vi "参数界面.vi"(8 "错误输入（无错误）":errorcluster, 10 "界面切换队列":refnum<queue>, 11 "VISA资源名称输入":refnum<visa-resource-name>) -> (0 "错误输出":errorcluster, 3 "VISA资源名称输出":refnum<visa-resource-name>)   [LabVIEW 2018]
panel:
  out "毫秒计时值":u32
  in  "枚举":T1(ring)
  in  "选项卡控件":enum32{"选项卡 1", "选项卡 2"}(tab)
  out "烧录座设定界面":bool
  out "极限参数界面":bool
  out "吸嘴偏移参数界面":bool
  out "读写R2481+R3禁用":bool
  out "DDT32534+R轴手动快速":dbl
  out "DDT32532+R轴手动慢速":dbl
  out "DDT32530+R轴减速时间":dbl
  out "DDT32528+R加速时间":dbl
  out "DDT32526+R轴最高速度":dbl
  out "DDT32524+R轴初始速度":dbl
  out "DDT32522+Z轴手动快速度":dbl
  out "DDT32520+Z轴手动慢速":dbl
  out "DDT32518+Z轴减速时间":dbl
  out "DDT32516+Z轴加速时间":dbl
  out "DDT32514+Z轴最高速度":dbl
  out "DDT32512+Z轴初始速度":dbl
  out "DDT32310+Y轴手动快速":dbl
  out "DDT32308+Y轴手动慢速":dbl
  out "DDT32306+Y轴减速时间":dbl
  out "DDT32304+Y轴加速时间":dbl
  out "DDT32302+Y轴最高速度":dbl
  out "DDT32300+Y轴初始速度":dbl
  out "DDT32510+X轴手动快速":dbl
  out "DDT32508+X轴手动慢速":dbl
  out "DDT32506+X轴减速时间":dbl
  out "DDT32504+X轴加速时间":dbl
  out "DDT32502+X轴最高速度":dbl
  out "DDT32500+X轴初始速度":dbl
  out "DDT32538+Z轴取料返回慢速长度":dbl
  out "DDT90356":dbl
  out "DDT90348":dbl
  out "自动界面":bool
  out "手动界面":bool
  out "参数界面":bool
  out "IO界面":bool
  out "产品界面":bool
  out "字符串":string
  out "DDT90352":dbl
  out "DDT90360":dbl
  out "DT1184":T2(ring)
  out "DDT32536+Z轴取料返回慢速":dbl
  in  "DT32730+枚举":enum16{"1拖2模式", "1拖4模式", "1拖8模式"}(ring)
  out "通讯周期":dbl
  # "X"
  # "Z1"
  # "XXXXX自动化设备有限公司"
  # "Z2"
  # "Y"
  # "速度参数"
  # "Z轴取料返回慢速长度"
  # "Z轴取料返回慢速"
  # "初始速度"
  # "最高速度"
  # "加速时间"
  # "减速时间"
  # "手动慢速"
  # "手动快速"
  # "X轴"
  # "Y轴"
  # "Z轴"
  # "R轴"
  # "选择1拖4或1拖8模式时，烧录座只能选择分开取放"
  # "烧录座模式请根据机器实际结构来更改，否则会出故障"
  # "烧录座模式"
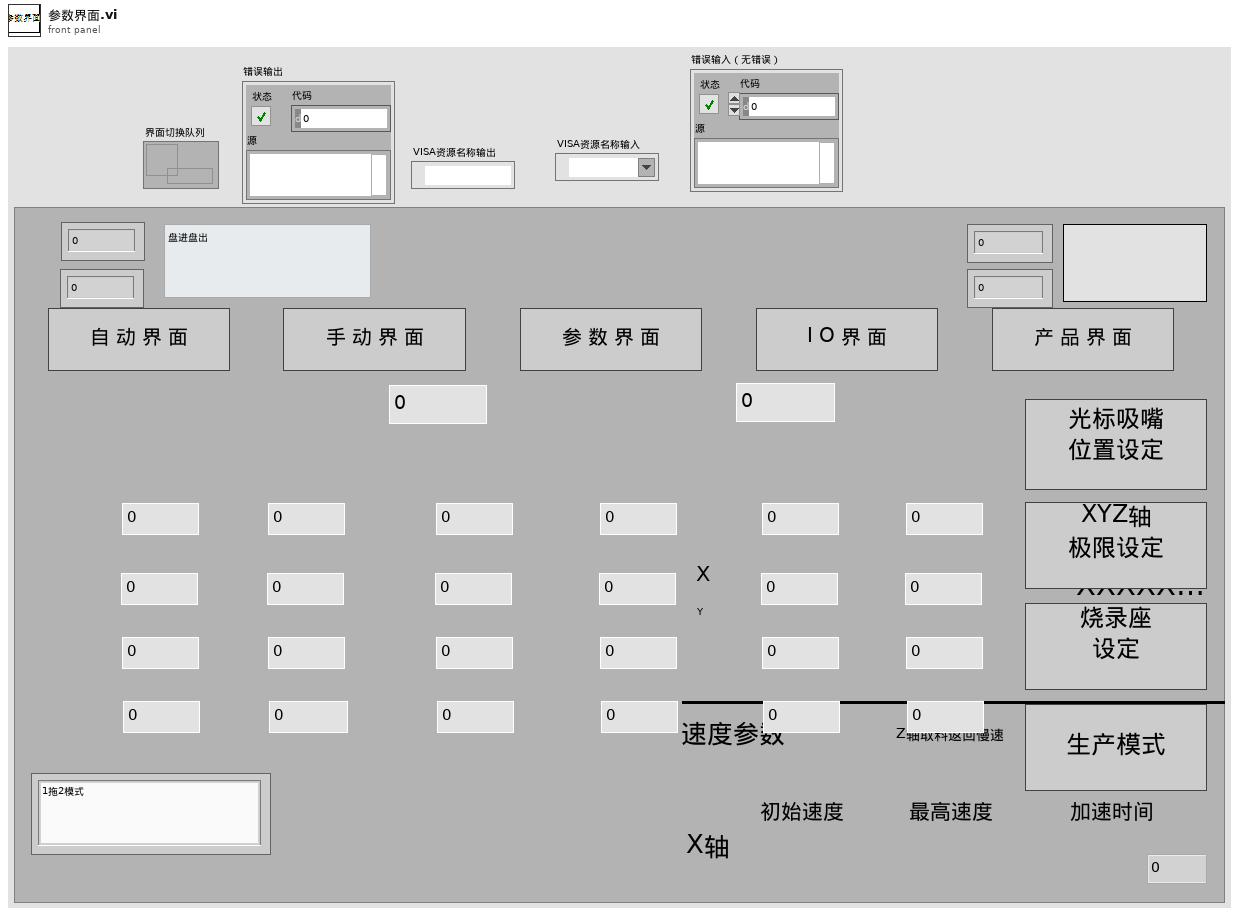
[diagram p1: front panel]
types:
  T1 = enum16{"读初始化", "读R3", "读R2481", "读DT32730+10", "读DDT32310+5", "读DDT32530+5", "读DDT32520+5", "读DDT32510+5", "读DDT32500+5", "读DDT32300+5", "读DDT90356", "读DT1184", "读DDT90348", ""}
  T2 = enum16{"盘进盘出", "卷进卷出", "盘进卷出", "管进盘出", "管进卷出", "卷进盘出", ""}
  T3 = enum8{"Enabled", "Disabled", "Disabled and Grayed Out"}
  T4 = typedef "数据簇.ctl" = cluster{"字符串":string, "数值":i32, "布尔":bool}
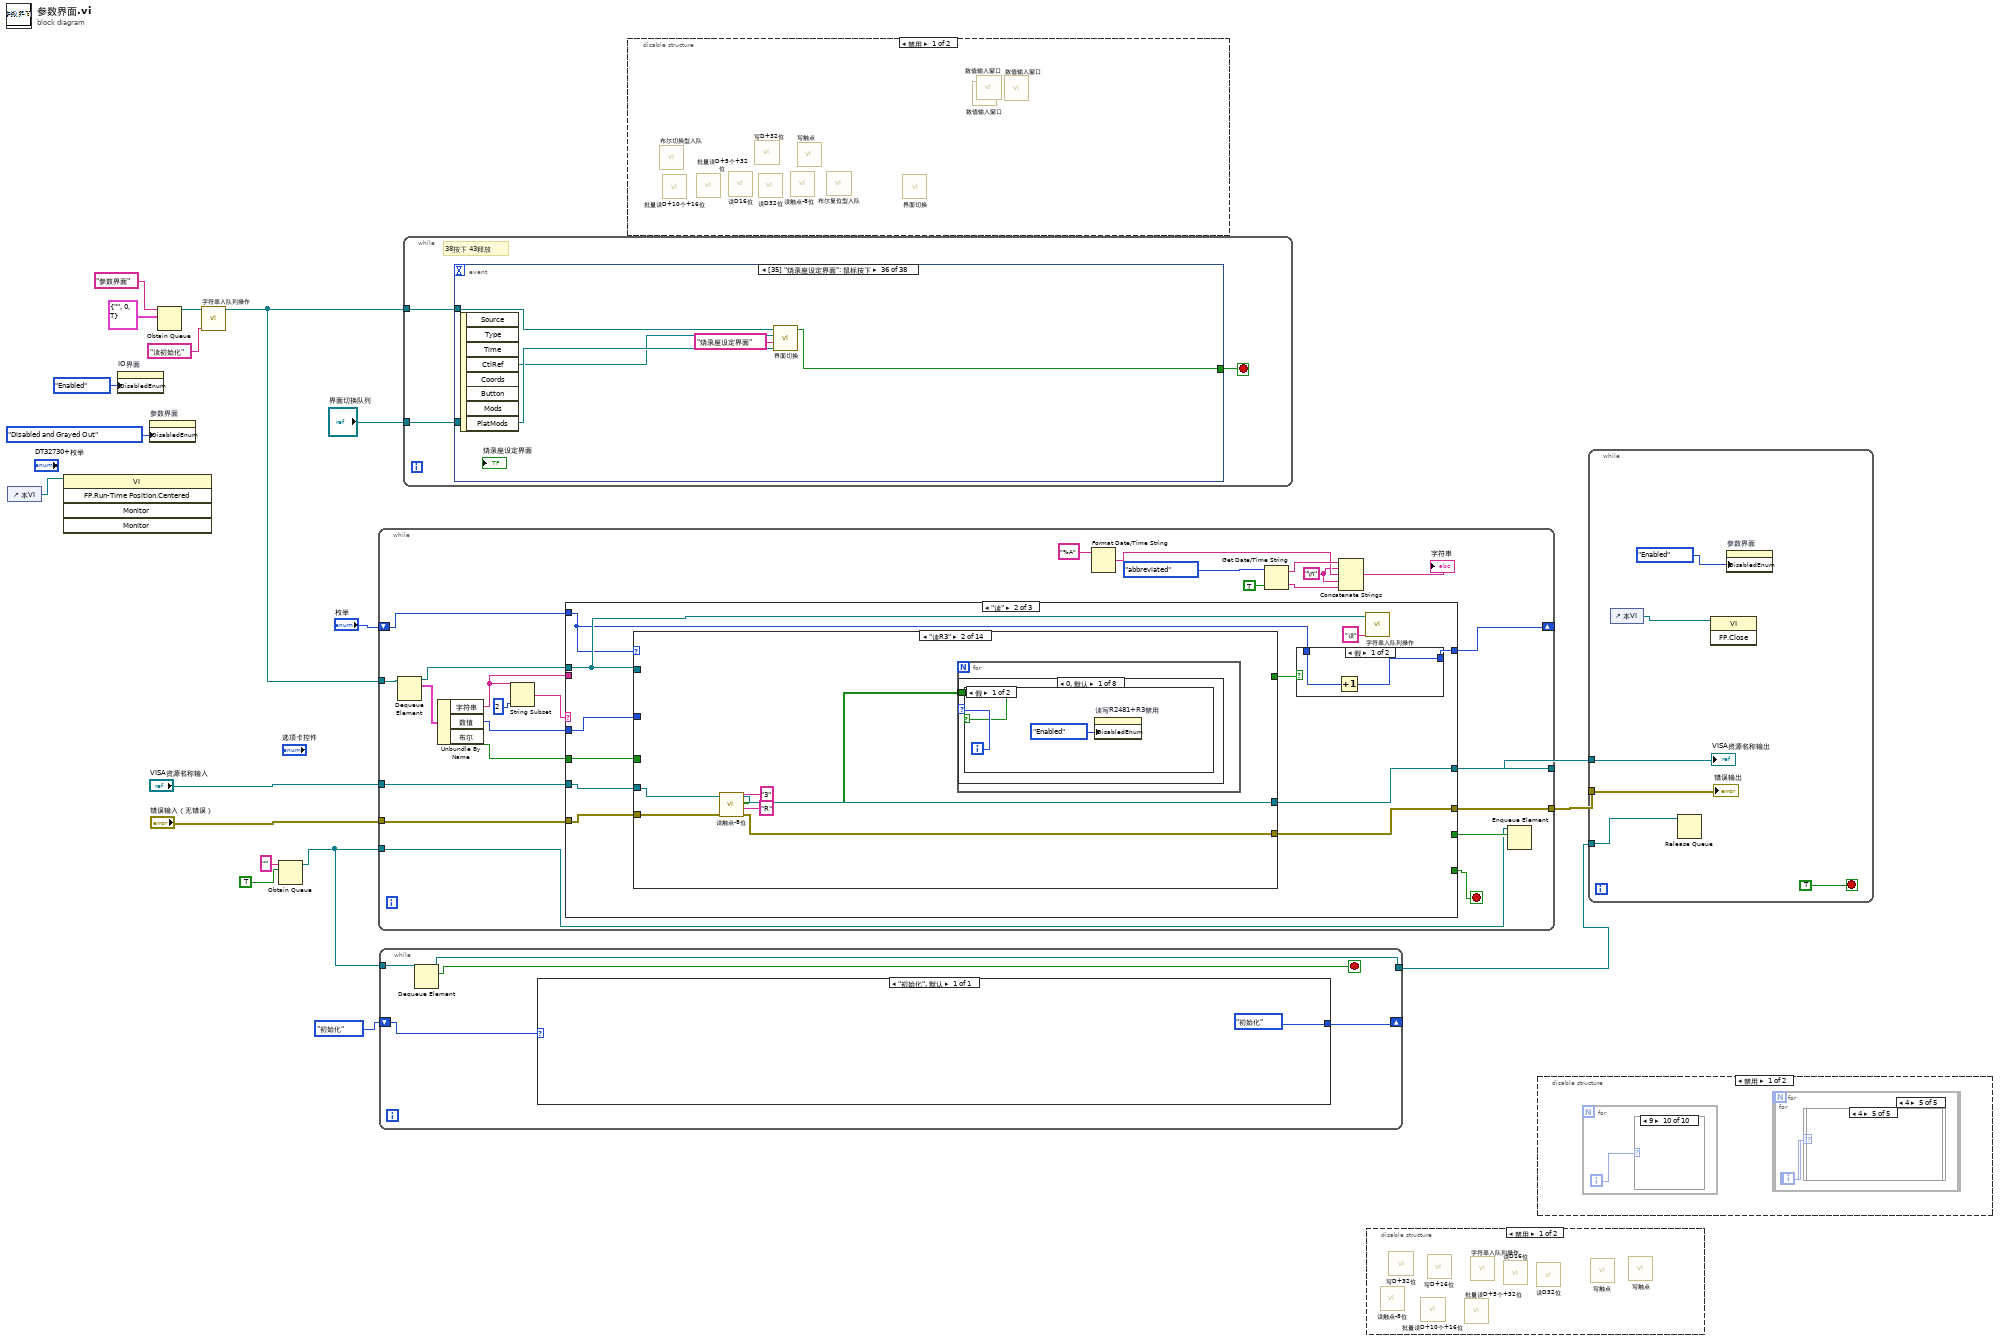
[diagram p0: block diagram]
diagram:
  n1 = control-ref of="本VI"() -> (w3:refnum<vi>)
  n2 = invoke class="VI" method="FP.Run-Time Position.Centered"(reference=w3) -> ()  [unwired: 4 in, 5 out]
  n3 = property on="IO界面" class="Bool"("DisabledEnum"=T3."Enabled" ("禁用")) -> ()  [unwired: 2 in, 2 out]
  n4 = property on="参数界面" class="Bool"("DisabledEnum"=T3."Disabled and Grayed Out" ("禁用")) -> ()  [unwired: 2 in, 2 out]
  n5 = Obtain Queue(name (unnamed)="参数界面" ("名称（未命名）"), element data type=T4 {"字符串"="", "数值"=0, "布尔"=TRUE}) -> (queue out=w12:refnum<queue>)  [unwired: 3 in, 2 out]
  n6 = call "字符串入队列操作.vi"("字符消息入队列"="读初始化", "界面切换队列"=w12) -> ("队列输出"=w4:refnum<queue>)  [unwired: 9 in]
  n7 = Obtain Queue(name (unnamed)="" ("名称（未命名）"), element data type=TRUE) -> (queue out=w7:refnum<queue>)  [unwired: 3 in, 2 out]
  n8 = while {
    tunnel: w4 -> [w40]
    tunnel: "VISA资源名称输入" -> [w33]
    tunnel: "错误输入（无错误）" -> [w32]
    tunnel: [w31] -> w14
    tunnel: [w30] -> w13
    shift-right: [w27] -> _
    shift-left: "枚举" -> [w28]
    tunnel: w7 -> [w20]
    stop <- w22 stop-if-true
    w24 = "\n"
    n9 = Dequeue Element(queue=w40) -> (queue out=w37:refnum<queue>, element=w39:T4)  [unwired: 2 in, 2 out]
    n10 = Unbundle By Name(w39) -> ("字符串"=w34:string, "数值"=w36:i32, "布尔"=w35:bool)
    n11 = String Subset(string=w34, length (rest)=2 ("长度（剩余）")) -> (substring=w38:string)  [unwired: 1 in]
    n12 = case shown="\"读\"" w38 {
      selector: w38 -> [w47 _ _]
      tunnel: w37 -> [_ w55 w231]
      tunnel: w36 -> [_ w62 w230]
      tunnel: w35 -> [_ w61 w229]
      tunnel: w34 -> [_ _ w223]
      tunnel: w33 -> [w46 w60 w228]
      tunnel: w32 -> [w45 w59 w227]
      tunnel: [w46 w58 w225] -> w31
      tunnel: [w45 w57 w224] -> w30
      tunnel: [_ _ w226] -> w22
      tunnel: w28 -> [_ w53 _]
      tunnel: [_ w52 _] -> w27
      tunnel: [_ _ w221] -> w21
      frame "", Default {
        n13 = Concatenate Strings("无对应消息分支**" ("消息"), w47, "**" ("字符串"), "读写状态机" ("字符串")) -> (w49:string)
        n14 = One Button Dialog(message=w49) -> ()  [unwired: 1 in, 1 out]
      }
      frame "读" {
        n15 = case shown="\"读R3\"" w53 {
          tunnel: w55 -> [_ _ _ _ _ _ _ _ _ _ _ _ _ _]
          tunnel: w62 -> [_ _ _ _ _ _ _ _ _ _ _ _ _ _]
          tunnel: w60 -> [w67 w74 w86 w95 w104 w113 w128 w141 w154 w167 w186 w195 w208 w220]
          tunnel: w59 -> [w66 w73 w85 w94 w103 w112 w127 w140 w153 w166 w185 w194 w207 w219]
          tunnel: [w67 w70 w82 w92 w101 w111 w126 w138 w151 w165 w184 w193 w206 w220] -> w58
          tunnel: [w66 w69 w81 w91 w100 w110 w125 w137 w150 w164 w183 w192 w205 w219] -> w57
          tunnel: w61 -> [_ _ _ _ _ _ _ _ _ _ _ _ _ _]
          tunnel: [_ _ _ _ _ _ _ _ _ _ _ _ _ TRUE] -> w54
          frame "读初始化" {
            n16 = Tick Count (ms)() -> (millisecond timer value=→"毫秒计时值":u32)
          }
          frame "读R3" {
            n17 = call "读触点-8位.vi"("error out"=w73, "触点类型"="R", "读取起始地址"="3", "VISA resource name out"=w74) -> ("error IO"=w69:errorcluster, "读取布尔数组"=w68:bool[], "VISA resource name out 2"=w70:refnum<visa-resource-name>)  [unwired: 4 in, 1 out]
            n18 = for {
              tunnel: w68 -> [w75] mode=indexing
              i -> [w76]
              n19 = case shown="0, 默认" w76 {
                tunnel: w75 -> [w77 _ _ _ _ _ _ _]
                frame 0, Default {
                  n20 = case shown="假" w77 {
                    frame False {
                      n21 = property on="读写R2481+R3禁用" class="Bool"("DisabledEnum"=T3."Enabled" ("禁用")) -> ()  [unwired: 2 in, 2 out]
                    }
                    frame True {
                      n22 = property on="读写R2481+R3禁用" class="Bool"("DisabledEnum"=T3."Disabled and Grayed Out" ("禁用")) -> ()  [unwired: 2 in, 2 out]
                    }
                  }
                }
                frame 1 {
                }
                frame 2 {
                }
                frame 3 {
                }
                frame 4 {
                }
                frame 5 {
                }
                frame 6 {
                }
                frame 7 {
                }
              }
            }
          }
          frame "读R2481" {
            n23 = call "读触点-8位.vi"("error out"=w85, "触点类型"="R", "读取起始地址"="2481", "VISA resource name out"=w86) -> ("error IO"=w81:errorcluster, "读取布尔数组"=w80:bool[], "VISA resource name out 2"=w82:refnum<visa-resource-name>)  [unwired: 4 in, 1 out]
            n24 = for {
              tunnel: w80 -> [w87] mode=indexing
              i -> [w88]
              n25 = case shown="0, 默认" w88 {
                tunnel: w87 -> [w89 _ _ _ _ _ _ _]
                frame 0, Default {
                  "读写R2481+R3禁用" <- w89
                }
                frame 1 {
                }
                frame 2 {
                }
                frame 3 {
                }
                frame 4 {
                }
                frame 5 {
                }
                frame 6 {
                }
                frame 7 {
                }
              }
            }
          }
          frame "读DT32730+10" {
            n26 = call "批量读D+10个+16位.vi"("error out"=w94, "读取D地址"=32730, "VISA resource name out"=w95) -> ("error IO"=w91:errorcluster, "数组"=w90:i32[], "VISA resource name out 2"=w92:refnum<visa-resource-name>)  [unwired: 5 in, 1 out]
            n27 = for {
              tunnel: w90 -> [w96] mode=indexing
              i -> [w97]
              n28 = case shown="0, 默认" w97 {
                tunnel: w96 -> [w98 _ _ _ _ _ _ _ _ _]
                frame 0, Default {
                  n29 = local write "DT32730+枚举"(w98) -> ()
                }
                frame 8 {
                }
                frame 9 {
                }
                frame 1 {
                }
                frame 2 {
                }
                frame 3 {
                }
                frame 4 {
                }
                frame 5 {
                }
                frame 6 {
                }
                frame 7 {
                }
              }
            }
          }
          frame "读DDT32310+5" {
            n30 = call "批量读D+5个+32位.vi"("error out"=w103, "读取D地址"=32310, "VISA resource name out"=w104) -> ("error IO"=w100:errorcluster, "数组"=w99:i32[], "VISA resource name out 2"=w101:refnum<visa-resource-name>)  [unwired: 5 in, 1 out]
            n31 = for {
              tunnel: w99 -> [w105] mode=indexing
              i -> [w106]
              n32 = case shown="0, 默认" w106 {
                tunnel: w105 -> [w107 _ _ _ _]
                frame 0, Default {
                  "DDT32310+Y轴手动快速" <- w107
                }
                frame 1 {
                }
                frame 2 {
                }
                frame 3 {
                }
                frame 4 {
                }
              }
            }
          }
          frame "读DDT32530+5" {
            n33 = call "批量读D+5个+32位.vi"("error out"=w112, "读取D地址"=32530, "VISA resource name out"=w113) -> ("error IO"=w110:errorcluster, "数组"=w108:i32[], "VISA resource name out 2"=w111:refnum<visa-resource-name>)  [unwired: 5 in, 1 out]
            n34 = for {
              tunnel: w108 -> [w114] mode=indexing
              i -> [w115]
              n35 = case shown="1" w115 {
                tunnel: w114 -> [w116 w117 w118 w119 w121]
                frame 0, Default {
                  "DDT32530+R轴减速时间" <- w116
                }
                frame 1 {
                  "DDT32532+R轴手动慢速" <- w117
                }
                frame 2 {
                  "DDT32534+R轴手动快速" <- w118
                }
                frame 3 {
                  "DDT32536+Z轴取料返回慢速" <- w119
                }
                frame 4 {
                  n36 = Divide(x=w121, y=100) -> (x/y=→"DDT32538+Z轴取料返回慢速长度":dbl)
                }
              }
            }
          }
          frame "读DDT32520+5" {
            n37 = call "批量读D+5个+32位.vi"("error out"=w127, "读取D地址"=32520, "VISA resource name out"=w128) -> ("error IO"=w125:errorcluster, "数组"=w123:i32[], "VISA resource name out 2"=w126:refnum<visa-resource-name>)  [unwired: 5 in, 1 out]
            n38 = for {
              tunnel: w123 -> [w129] mode=indexing
              i -> [w130]
              n39 = case shown="0, 默认" w130 {
                tunnel: w129 -> [w131 w132 w133 w134 w135]
                frame 0, Default {
                  "DDT32520+Z轴手动慢速" <- w131
                }
                frame 1 {
                  "DDT32522+Z轴手动快速度" <- w132
                }
                frame 2 {
                  "DDT32524+R轴初始速度" <- w133
                }
                frame 3 {
                  "DDT32526+R轴最高速度" <- w134
                }
                frame 4 {
                  "DDT32528+R加速时间" <- w135
                }
              }
            }
          }
          frame "读DDT32510+5" {
            n40 = call "批量读D+5个+32位.vi"("error out"=w140, "读取D地址"=32510, "VISA resource name out"=w141) -> ("error IO"=w137:errorcluster, "数组"=w136:i32[], "VISA resource name out 2"=w138:refnum<visa-resource-name>)  [unwired: 5 in, 1 out]
            n41 = for {
              tunnel: w136 -> [w142] mode=indexing
              i -> [w143]
              n42 = case shown="4" w143 {
                tunnel: w142 -> [w144 w145 w146 w147 w148]
                frame 0, Default {
                  "DDT32510+X轴手动快速" <- w144
                }
                frame 1 {
                  "DDT32512+Z轴初始速度" <- w145
                }
                frame 2 {
                  "DDT32514+Z轴最高速度" <- w146
                }
                frame 3 {
                  "DDT32516+Z轴加速时间" <- w147
                }
                frame 4 {
                  "DDT32518+Z轴减速时间" <- w148
                }
              }
            }
          }
          frame "读DDT32500+5" {
            n43 = call "批量读D+5个+32位.vi"("error out"=w153, "读取D地址"=32500, "VISA resource name out"=w154) -> ("error IO"=w150:errorcluster, "数组"=w149:i32[], "VISA resource name out 2"=w151:refnum<visa-resource-name>)  [unwired: 5 in, 1 out]
            n44 = for {
              tunnel: w149 -> [w155] mode=indexing
              i -> [w156]
              n45 = case shown="4" w156 {
                tunnel: w155 -> [w157 w158 w159 w160 w161]
                frame 0, Default {
                  "DDT32500+X轴初始速度" <- w157
                }
                frame 1 {
                  "DDT32502+X轴最高速度" <- w158
                }
                frame 2 {
                  "DDT32504+X轴加速时间" <- w159
                }
                frame 3 {
                  "DDT32506+X轴减速时间" <- w160
                }
                frame 4 {
                  "DDT32508+X轴手动慢速" <- w161
                }
              }
            }
          }
          frame "读DDT32300+5" {
            n46 = call "批量读D+5个+32位.vi"("error out"=w166, "读取D地址"=32300, "VISA resource name out"=w167) -> ("error IO"=w164:errorcluster, "数组"=w162:i32[], "VISA resource name out 2"=w165:refnum<visa-resource-name>)  [unwired: 5 in, 1 out]
            n47 = for {
              tunnel: w162 -> [w168] mode=indexing
              i -> [w169]
              n48 = case shown="0, 默认" w169 {
                tunnel: w168 -> [w170 w171 w172 w173 w174]
                frame 0, Default {
                  "DDT32300+Y轴初始速度" <- w170
                }
                frame 1 {
                  "DDT32302+Y轴最高速度" <- w171
                }
                frame 2 {
                  "DDT32304+Y轴加速时间" <- w172
                }
                frame 3 {
                  "DDT32306+Y轴减速时间" <- w173
                }
                frame 4 {
                  "DDT32308+Y轴手动慢速" <- w174
                }
              }
            }
          }
          frame "读DDT90356" {
            n49 = call "批量读D+5个+32位.vi"("error out"=w185, "读取D地址"=90356, "VISA resource name out"=w186) -> ("error IO"=w183:errorcluster, "数组"=w189:i32[], "VISA resource name out 2"=w184:refnum<visa-resource-name>)  [unwired: 5 in, 1 out]
            n50 = Index Array(array=w189, index #1=0 ("索引"), index #2=2 ("索引")) -> (element #1=w182:i32, element #2=w181:i32)
            n51 = To Double Precision Float(number=w182) -> (double precision float=w180:dbl)
            n52 = To Double Precision Float(number=w181) -> (double precision float=w177:dbl)
            n53 = Divide(x=w180, y=100.0) -> (x/y=→"DDT90356":dbl)
            n54 = Divide(x=w177, y=100.0) -> (x/y=→"DDT90360":dbl)
          }
          frame "读DT1184" {
            n55 = call "读D16位.vi"("error out"=w194, "读取D地址"=1184, "VISA resource name out"=w195) -> ("error IO"=w192:errorcluster, "数值"=→"DT1184":u32, "VISA resource name out 2"=w193:refnum<visa-resource-name>)  [unwired: 5 in, 1 out]
          }
          frame "读DDT90348" {
            n56 = call "批量读D+5个+32位.vi"("error out"=w207, "读取D地址"=90348, "VISA resource name out"=w208) -> ("error IO"=w205:errorcluster, "数组"=w212:i32[], "VISA resource name out 2"=w206:refnum<visa-resource-name>)  [unwired: 5 in, 1 out]
            n57 = Index Array(array=w212, index #1=0 ("索引"), index #2=2 ("索引")) -> (element #1=w204:i32, element #2=w203:i32)
            n58 = To Double Precision Float(number=w204) -> (double precision float=w202:dbl)
            n59 = To Double Precision Float(number=w203) -> (double precision float=w198:dbl)
            n60 = Divide(x=w202, y=100.0) -> (x/y=→"DDT90348":dbl)
            n61 = Divide(x=w198, y=100.0) -> (x/y=→"DDT90352":dbl)
          }
          frame "" {
            n62 = local read "毫秒计时值"() -> (w216:u32)
            n63 = Tick Count (ms)() -> (millisecond timer value=w217:u32)
            n64 = Subtract(x=w217, y=w216) -> (x-y=w215:u32)
            n65 = Divide(x=w215, y=u32 1000) -> (x/y=→"通讯周期":dbl)
          }
        }
        n66 = case shown="假" w54 {
          tunnel: w53 -> [w64 _]
          tunnel: [w63 _] -> w52
          frame False {
            n67 = Increment(x=w64) -> (x+1=w63:T1)
          }
          frame True {
          }
        }
        n68 = call "字符串入队列操作.vi"("字符消息入队列"="读", "界面切换队列"=w55) -> ()  [unwired: 9 in, 1 out]
      }
      frame "写" {
        n69 = call "状态匹配.vi"("输入状态"=w223) -> ("输出状态"=w222:string)  [unwired: 10 in]
        n70 = case shown="\"写DDT\"" w222 {
          selector: w222 -> [w234 _ _ _ _]
          tunnel: w231 -> [_ _ _ _ w274]
          tunnel: w230 -> [_ w240 w257 _ _]
          tunnel: w229 -> [_ _ _ w268 _]
          tunnel: w228 -> [w233 w250 w261 w273 w279]
          tunnel: w227 -> [w232 w249 w260 w272 w278]
          tunnel: [_ _ _ _ w277] -> w226
          tunnel: [w233 w248 w259 w271 w279] -> w225
          tunnel: [w232 w247 w258 w270 w278] -> w224
          tunnel: w223 -> [_ w239 w251 w262 _]
          tunnel: [_ _ _ _ w277] -> w221
          frame "", Default {
            n71 = Concatenate Strings("无对应消息分支**" ("消息"), w234, "**" ("字符串"), "写状态机" ("字符串")) -> (w238:string)
            n72 = One Button Dialog(message=w238) -> ()  [unwired: 1 in, 1 out]
          }
          frame "写DT" {
            n73 = String Length(string=w239) -> (length=w245:i32)
            n74 = Subtract(x=w245, y=4) -> (x-y=w243:i32)
            n75 = String Subset(string=w239, offset (0)=4 ("偏移量(0)"), length (rest)=w243) -> (substring=w242:string)
            n76 = Decimal String To Number(string=w242) -> (number=w241:i32)  [unwired: 2 in, 1 out]
            n77 = call "写D+16位.vi"("error out"=w249, "输入数值"=w240, "输入地址D"=w241, "VISA resource name out"=w250) -> ("error out 2"=w247:errorcluster, "VISA resource name out 2"=w248:refnum<visa-resource-name>)  [unwired: 3 in, 3 out]
          }
          frame "写DDT" {
            n78 = String Length(string=w251) -> (length=w255:i32)
            n79 = Subtract(x=w255, y=5) -> ()  [unwired: 1 out]
            n80 = String Subset(string=w251, offset (0)=5 ("偏移量(0)")) -> (substring=w252:string)  [unwired: 1 in]
            n81 = Decimal String To Number(string=w252) -> (number=w253:i32)  [unwired: 2 in, 1 out]
            n82 = call "写D+32位.vi"("error out"=w260, "输入数值"=w257, "输入地址D"=w253, "VISA resource name out"=w261) -> ("error out 2"=w258:errorcluster, "VISA resource name out 2"=w259:refnum<visa-resource-name>)  [unwired: 4 in, 2 out]
          }
          frame "写R" {
            n83 = String Length(string=w262) -> (length=w266:i32)
            n84 = Subtract(x=w266, y=3) -> (x-y=w264:i32)
            n85 = String Subset(string=w262, offset (0)=3 ("偏移量(0)"), length (rest)=w264) -> (substring=w263:string)
            n86 = call "写触点.vi"("布尔"=w268, "error out"=w272, "触点类型"="R", "写入起始地址"=w263, "VISA resource name out"=w273) -> ("error IO"=w270:errorcluster, "VISA resource name out 2"=w271:refnum<visa-resource-name>)  [unwired: 4 in, 1 out]
          }
          frame "写退出" {
            w277 = TRUE
            n87 = Flush Queue(queue=w274) -> (queue out=w275:refnum<queue>, error out=w276:errorcluster)  [unwired: 1 in, 1 out]
            n88 = Release Queue(queue=w275, error in (no error)=w276) -> ()  [unwired: 1 in, 3 out]
          }
        }
      }
    }
    n89 = Format Date/Time String(time format string (%c)="%A" ("时间格式字符串(%c)")) -> (date/time string=w25:string)  [unwired: 2 in]
    n90 = Get Date/Time String(date format (0)=enum16{"short", "long", "abbreviated"}."abbreviated" ("日期格式(0)"), want seconds? (F)=TRUE ("需要秒？(F)")) -> (date string=w42:string, time string=w23:string)  [unwired: 1 in]
    n91 = Concatenate Strings(w42, w24, w25, w24, w23) -> (→"字符串":string)
    n92 = Enqueue Element(queue=w20, element=w21) -> ()  [unwired: 2 in, 3 out]
  }
  n93 = while {
    shift-right: [w283] -> _
    shift-left: enum16{"初始化"}."初始化" -> [w284]
    tunnel: w7 -> [w282]
    tunnel: [w280] -> w6
    stop <- w281 stop-if-true
    n94 = Dequeue Element(queue=w282) -> (queue out=w280:refnum<queue>, element=w281:bool)  [unwired: 2 in, 2 out]
    n95 = case shown="\"初始化\", 默认" w284 {
      tunnel: [enum16{"初始化"}."初始化"] -> w283
      frame "初始化", Default {
      }
    }
  }
  n96 = while {
    tunnel: w4 -> [w287]
    tunnel: "界面切换队列" -> [w286]
    stop <- w288 stop-if-true
    # "38按下 43释放"
    n97 = event shown="[35] \"烧录座设定界面\": 鼠标按下" {
      selector: _ -> [_ _ _ _ _ _ _ _ _ _ _ _ _ _ _ _ _ _ _ _ _ _ _ _ _ _ _ _ _ _ _ _ _ _ _ _ _ _]
      dyn-events: _ -> [_ _ _ _ _ _ _ _ _ _ _ _ _ _ _ _ _ _ _ _ _ _ _ _ _ _ _ _ _ _ _ _ _ _ _ _ _ _]
      timeout: _ -> [_ _ _ _ _ _ _ _ _ _ _ _ _ _ _ _ _ _ _ _ _ _ _ _ _ _ _ _ _ _ _ _ _ _ _ _ _ _]
      tunnel: [w289 _ _ _ _ _ _ _ _ _ _ _ _ _ _ _ _ _ _ _ _ _ _ _ _ _ _ _ _ w509 w514 w523 w524 w529 w534 w539 _ w546] -> w288
      tunnel: w287 -> [w293 w297 w300 w308 w315 w324 w332 w340 w348 w356 w364 w372 w380 w388 w396 w404 w412 w420 w428 w436 w444 w452 w460 w468 w476 w484 w492 w500 w508 w513 w518 w522 w528 w533 w538 w543 _ w545]
      tunnel: w286 -> [w292 _ _ _ _ _ _ _ _ _ _ _ _ _ _ _ _ _ _ _ _ _ _ _ _ _ _ _ _ w512 w517 w521 w527 w532 w537 w542 _ w544]
      event "IO界面": Mouse Down {
        n98 = event-data() -> ("CtlRef"=w291:refnum<vi>)  [unwired: 1 in, 7 out]
        n99 = call "界面切换.vi"("界面切换队列输入"=w292, "切换界面名称输入"="IO界面", "Bool引用句柄"=w291, "状态转移输入"=w293) -> ("布尔"=w289:bool)  [unwired: 7 in]
      }
      event "读写R2481+R3禁用": Mouse Down {
        n100 = event-data() -> ("CtlRef"=w296:refnum<vi>)  [unwired: 1 in, 7 out]
        n101 = call "布尔切换型入队.vi"("字符串"="写R2481", "true启用入队"=TRUE, "控件引用"=w296, "消息入队列"=w297) -> ()  [unwired: 8 in]
      }
      event "DT32730+枚举": Value Change {
        n102 = event-data() -> ("NewVal"=w299:enum16{"1拖2模式", "1拖4模式", "1拖8模式"})  [unwired: 1 in, 5 out]
        n103 = call "字符串入队列操作.vi"("字符消息入队列"="写DT32730", "数值"=w299, "界面切换队列"=w300) -> ()  [unwired: 8 in, 1 out]
      }
      event "DDT32536+Z轴取料返回慢速": Mouse Down {
        n104 = event-data() -> ("CtlRef"=w301:refnum<vi>)  [unwired: 1 in, 7 out]
        n105 = call "数值输入窗口.vi"("消息入队"=w308, "字符串"="Z轴取料返回慢速", "字符消息入队列"="写DDT32536", "输入下限"=100.0, "输入上限"=60000.0, "转换比例"=u32 1, "数据类型"=enum16{"32位", "16位"}."32位", "控件引用"=w301) -> ()  [unwired: 5 in, 3 out]
      }
      event "DDT32538+Z轴取料返回慢速长度": Mouse Down {
        n106 = event-data() -> ("CtlRef"=w316:refnum<vi>)  [unwired: 1 in, 7 out]
        n107 = call "数值输入窗口.vi"("消息入队"=w315, "字符串"="Z轴取料返回慢速长度", "字符消息入队列"="写DDT32538", "输入下限"=0.0, "输入上限"=1000.0, "转换比例"=u32 100, "数据类型"=enum16{"32位", "16位"}."32位", "控件引用"=w316) -> ()  [unwired: 5 in, 3 out]
      }
      event "DDT32500+X轴初始速度": Mouse Down {
        n108 = event-data() -> ("CtlRef"=w317:refnum<vi>)  [unwired: 1 in, 7 out]
        n109 = call "数值输入窗口.vi"("消息入队"=w324, "字符串"="X轴初始速度", "字符消息入队列"="写DDT32500", "输入下限"=100.0, "输入上限"=1000.0, "转换比例"=u32 1, "数据类型"=enum16{"32位", "16位"}."32位", "控件引用"=w317) -> ()  [unwired: 5 in, 3 out]
      }
      event "DDT32502+X轴最高速度": Mouse Down {
        n110 = event-data() -> ("CtlRef"=w325:refnum<vi>)  [unwired: 1 in, 7 out]
        n111 = call "数值输入窗口.vi"("消息入队"=w332, "字符串"="X轴最高速度", "字符消息入队列"="写DDT32502", "输入下限"=100.0, "输入上限"=99000.0, "转换比例"=u32 1, "数据类型"=enum16{"32位", "16位"}."32位", "控件引用"=w325) -> ()  [unwired: 5 in, 3 out]
      }
      event "DDT32504+X轴加速时间": Mouse Down {
        n112 = event-data() -> ("CtlRef"=w334:refnum<vi>)  [unwired: 1 in, 7 out]
        n113 = call "数值输入窗口.vi"("消息入队"=w340, "字符串"="X轴加速时间", "字符消息入队列"="写DDT32504", "输入下限"=100.0, "输入上限"=99000.0, "转换比例"=u32 1, "数据类型"=enum16{"32位", "16位"}."32位", "控件引用"=w334) -> ()  [unwired: 5 in, 3 out]
      }
      event "DDT32506+X轴减速时间": Mouse Down {
        n114 = event-data() -> ("CtlRef"=w341:refnum<vi>)  [unwired: 1 in, 7 out]
        n115 = call "数值输入窗口.vi"("消息入队"=w348, "字符串"="X轴减速时间", "字符消息入队列"="写DDT32506", "输入下限"=100.0, "输入上限"=99000.0, "转换比例"=u32 1, "数据类型"=enum16{"32位", "16位"}."32位", "控件引用"=w341) -> ()  [unwired: 5 in, 3 out]
      }
      event "DDT32508+X轴手动慢速": Mouse Down {
        n116 = event-data() -> ("CtlRef"=w349:refnum<vi>)  [unwired: 1 in, 7 out]
        n117 = call "数值输入窗口.vi"("消息入队"=w356, "字符串"="X轴手动慢速", "字符消息入队列"="写DDT32508", "输入下限"=100.0, "输入上限"=99000.0, "转换比例"=u32 1, "数据类型"=enum16{"32位", "16位"}."32位", "控件引用"=w349) -> ()  [unwired: 5 in, 3 out]
      }
      event "DDT32510+X轴手动快速": Mouse Down {
        n118 = event-data() -> ("CtlRef"=w357:refnum<vi>)  [unwired: 1 in, 7 out]
        n119 = call "数值输入窗口.vi"("消息入队"=w364, "字符串"="X轴手动快速", "字符消息入队列"="写DDT32510", "输入下限"=100.0, "输入上限"=99000.0, "转换比例"=u32 1, "数据类型"=enum16{"32位", "16位"}."32位", "控件引用"=w357) -> ()  [unwired: 5 in, 3 out]
      }
      event "DDT32300+Y轴初始速度": Mouse Down {
        n120 = event-data() -> ("CtlRef"=w365:refnum<vi>)  [unwired: 1 in, 7 out]
        n121 = call "数值输入窗口.vi"("消息入队"=w372, "字符串"="Y轴初始速度", "字符消息入队列"="写DDT32300", "输入下限"=100.0, "输入上限"=1000.0, "转换比例"=u32 1, "数据类型"=enum16{"32位", "16位"}."32位", "控件引用"=w365) -> ()  [unwired: 5 in, 3 out]
      }
      event "DDT32302+Y轴最高速度": Mouse Down {
        n122 = event-data() -> ("CtlRef"=w373:refnum<vi>)  [unwired: 1 in, 7 out]
        n123 = call "数值输入窗口.vi"("消息入队"=w380, "字符串"="Y轴最高速度", "字符消息入队列"="写DDT32302", "输入下限"=100.0, "输入上限"=99000.0, "转换比例"=u32 1, "数据类型"=enum16{"32位", "16位"}."32位", "控件引用"=w373) -> ()  [unwired: 5 in, 3 out]
      }
      event "DDT32304+Y轴加速时间": Mouse Down {
        n124 = event-data() -> ("CtlRef"=w383:refnum<vi>)  [unwired: 1 in, 7 out]
        n125 = call "数值输入窗口.vi"("消息入队"=w388, "字符串"="Y轴加速时间", "字符消息入队列"="写DDT32304", "输入下限"=100.0, "输入上限"=99000.0, "转换比例"=u32 1, "数据类型"=enum16{"32位", "16位"}."32位", "控件引用"=w383) -> ()  [unwired: 5 in, 3 out]
      }
      event "DDT32306+Y轴减速时间": Mouse Down {
        n126 = event-data() -> ("CtlRef"=w389:refnum<vi>)  [unwired: 1 in, 7 out]
        n127 = call "数值输入窗口.vi"("消息入队"=w396, "字符串"="Y轴减速时间", "字符消息入队列"="写DDT32306", "输入下限"=100.0, "输入上限"=99000.0, "转换比例"=u32 1, "数据类型"=enum16{"32位", "16位"}."32位", "控件引用"=w389) -> ()  [unwired: 5 in, 3 out]
      }
      event "DDT32308+Y轴手动慢速": Mouse Down {
        n128 = event-data() -> ("CtlRef"=w397:refnum<vi>)  [unwired: 1 in, 7 out]
        n129 = call "数值输入窗口.vi"("消息入队"=w404, "字符串"="Y轴手动慢速", "字符消息入队列"="写DDT32308", "输入下限"=100.0, "输入上限"=99000.0, "转换比例"=u32 1, "数据类型"=enum16{"32位", "16位"}."32位", "控件引用"=w397) -> ()  [unwired: 5 in, 3 out]
      }
      event "DDT32310+Y轴手动快速": Mouse Down {
        n130 = event-data() -> ("CtlRef"=w405:refnum<vi>)  [unwired: 1 in, 7 out]
        n131 = call "数值输入窗口.vi"("消息入队"=w412, "字符串"="Y轴手动快速", "字符消息入队列"="写DDT32310", "输入下限"=100.0, "输入上限"=99000.0, "转换比例"=u32 1, "数据类型"=enum16{"32位", "16位"}."32位", "控件引用"=w405) -> ()  [unwired: 5 in, 3 out]
      }
      event "DDT32512+Z轴初始速度": Mouse Down {
        n132 = event-data() -> ("CtlRef"=w413:refnum<vi>)  [unwired: 1 in, 7 out]
        n133 = call "数值输入窗口.vi"("消息入队"=w420, "字符串"="Z轴初始速度", "字符消息入队列"="写DDT32512", "输入下限"=100.0, "输入上限"=1000.0, "转换比例"=u32 1, "数据类型"=enum16{"32位", "16位"}."32位", "控件引用"=w413) -> ()  [unwired: 5 in, 3 out]
      }
      event "DDT32514+Z轴最高速度": Mouse Down {
        n134 = event-data() -> ("CtlRef"=w421:refnum<vi>)  [unwired: 1 in, 7 out]
        n135 = call "数值输入窗口.vi"("消息入队"=w428, "字符串"="Z轴最高速度", "字符消息入队列"="写DDT32514", "输入下限"=100.0, "输入上限"=9900.0, "转换比例"=u32 1, "数据类型"=enum16{"32位", "16位"}."32位", "控件引用"=w421) -> ()  [unwired: 5 in, 3 out]
      }
      event "DDT32516+Z轴加速时间": Mouse Down {
        n136 = event-data() -> ("CtlRef"=w429:refnum<vi>)  [unwired: 1 in, 7 out]
        n137 = call "数值输入窗口.vi"("消息入队"=w436, "字符串"="Z轴加速时间", "字符消息入队列"="写DDT32516", "输入下限"=100.0, "输入上限"=99000.0, "转换比例"=u32 1, "数据类型"=enum16{"32位", "16位"}."32位", "控件引用"=w429) -> ()  [unwired: 5 in, 3 out]
      }
      event "DDT32518+Z轴减速时间": Mouse Down {
        n138 = event-data() -> ("CtlRef"=w437:refnum<vi>)  [unwired: 1 in, 7 out]
        n139 = call "数值输入窗口.vi"("消息入队"=w444, "字符串"="Z轴减速时间", "字符消息入队列"="写DDT32518", "输入下限"=100.0, "输入上限"=99000.0, "转换比例"=u32 1, "数据类型"=enum16{"32位", "16位"}."32位", "控件引用"=w437) -> ()  [unwired: 5 in, 3 out]
      }
      event "DDT32520+Z轴手动慢速": Mouse Down {
        n140 = event-data() -> ("CtlRef"=w445:refnum<vi>)  [unwired: 1 in, 7 out]
        n141 = call "数值输入窗口.vi"("消息入队"=w452, "字符串"="Z轴手动慢速", "字符消息入队列"="写DDT32520", "输入下限"=100.0, "输入上限"=99000.0, "转换比例"=u32 1, "数据类型"=enum16{"32位", "16位"}."32位", "控件引用"=w445) -> ()  [unwired: 5 in, 3 out]
      }
      event "DDT32522+Z轴手动快速度": Mouse Down {
        n142 = event-data() -> ("CtlRef"=w453:refnum<vi>)  [unwired: 1 in, 7 out]
        n143 = call "数值输入窗口.vi"("消息入队"=w460, "字符串"="Z轴手动快速", "字符消息入队列"="写DDT32522", "输入下限"=100.0, "输入上限"=99900.0, "转换比例"=u32 1, "数据类型"=enum16{"32位", "16位"}."32位", "控件引用"=w453) -> ()  [unwired: 5 in, 3 out]
      }
      event "DDT32524+R轴初始速度": Mouse Down {
        n144 = event-data() -> ("CtlRef"=w461:refnum<vi>)  [unwired: 1 in, 7 out]
        n145 = call "数值输入窗口.vi"("消息入队"=w468, "字符串"="R轴初始速度", "字符消息入队列"="写DDT32524", "输入下限"=100.0, "输入上限"=1000.0, "转换比例"=u32 1, "数据类型"=enum16{"32位", "16位"}."32位", "控件引用"=w461) -> ()  [unwired: 5 in, 3 out]
      }
      event "DDT32526+R轴最高速度": Mouse Down {
        n146 = event-data() -> ("CtlRef"=w469:refnum<vi>)  [unwired: 1 in, 7 out]
        n147 = call "数值输入窗口.vi"("消息入队"=w476, "字符串"="R轴最高速度", "字符消息入队列"="写DDT32526", "输入下限"=100.0, "输入上限"=9900.0, "转换比例"=u32 1, "数据类型"=enum16{"32位", "16位"}."32位", "控件引用"=w469) -> ()  [unwired: 5 in, 3 out]
      }
      event "DDT32528+R加速时间": Mouse Down {
        n148 = event-data() -> ("CtlRef"=w477:refnum<vi>)  [unwired: 1 in, 7 out]
        n149 = call "数值输入窗口.vi"("消息入队"=w484, "字符串"="R轴加速时间", "字符消息入队列"="写DDT32528", "输入下限"=100.0, "输入上限"=99900.0, "转换比例"=u32 1, "数据类型"=enum16{"32位", "16位"}."32位", "控件引用"=w477) -> ()  [unwired: 5 in, 3 out]
      }
      event "DDT32530+R轴减速时间": Mouse Down {
        n150 = event-data() -> ("CtlRef"=w487:refnum<vi>)  [unwired: 1 in, 7 out]
        n151 = call "数值输入窗口.vi"("消息入队"=w492, "字符串"="R轴减速时间", "字符消息入队列"="写DDT32530", "输入下限"=100.0, "输入上限"=99000.0, "转换比例"=u32 1, "数据类型"=enum16{"32位", "16位"}."32位", "控件引用"=w487) -> ()  [unwired: 5 in, 3 out]
      }
      event "DDT32532+R轴手动慢速": Mouse Down {
        n152 = event-data() -> ("CtlRef"=w495:refnum<vi>)  [unwired: 1 in, 7 out]
        n153 = call "数值输入窗口.vi"("消息入队"=w500, "字符串"="R轴手动慢速", "字符消息入队列"="写DDT32532", "输入下限"=100.0, "输入上限"=99000.0, "转换比例"=u32 1, "数据类型"=enum16{"32位", "16位"}."32位", "控件引用"=w495) -> ()  [unwired: 5 in, 3 out]
      }
      event "DDT32534+R轴手动快速": Mouse Down {
        n154 = event-data() -> ("CtlRef"=w501:refnum<vi>)  [unwired: 1 in, 7 out]
        n155 = call "数值输入窗口.vi"("消息入队"=w508, "字符串"="R轴手动快速", "字符消息入队列"="写DDT32534", "输入下限"=100.0, "输入上限"=99900.0, "转换比例"=u32 1, "数据类型"=enum16{"32位", "16位"}."32位", "控件引用"=w501) -> ()  [unwired: 5 in, 3 out]
      }
      event "参数界面": Mouse Down {
        n156 = event-data() -> ("CtlRef"=w511:refnum<vi>)  [unwired: 1 in, 7 out]
        n157 = call "界面切换.vi"("界面切换队列输入"=w512, "切换界面名称输入"="参数界面", "Bool引用句柄"=w511, "状态转移输入"=w513) -> ("布尔"=w509:bool)  [unwired: 7 in]
      }
      event "产品界面": Mouse Down {
        n158 = event-data() -> ("CtlRef"=w516:refnum<vi>)  [unwired: 1 in, 7 out]
        n159 = call "界面切换.vi"("界面切换队列输入"=w517, "切换界面名称输入"="产品界面", "Bool引用句柄"=w516, "状态转移输入"=w518) -> ("布尔"=w514:bool)  [unwired: 7 in]
      }
      event "手动界面": Mouse Down {
        n160 = event-data() -> ("CtlRef"=w520:refnum<vi>)  [unwired: 1 in, 7 out]
        n161 = call "界面切换.vi"("界面切换队列输入"=w521, "切换界面名称输入"="手动界面", "Bool引用句柄"=w520, "状态转移输入"=w522) -> ("布尔"=w523:bool)  [unwired: 7 in]
      }
      event "自动界面": Mouse Down {
        n162 = event-data() -> ("CtlRef"=w526:refnum<vi>)  [unwired: 1 in, 7 out]
        n163 = call "界面切换.vi"("界面切换队列输入"=w527, "切换界面名称输入"="自动界面", "Bool引用句柄"=w526, "状态转移输入"=w528) -> ("布尔"=w524:bool)  [unwired: 7 in]
      }
      event "吸嘴偏移参数界面": Mouse Down {
        n164 = event-data() -> ("CtlRef"=w530:refnum<vi>)  [unwired: 1 in, 7 out]
        n165 = call "界面切换.vi"("界面切换队列输入"=w532, "切换界面名称输入"="吸嘴偏移参数界面", "Bool引用句柄"=w530, "状态转移输入"=w533) -> ("布尔"=w529:bool)  [unwired: 7 in]
      }
      event "极限参数界面": Mouse Down {
        n166 = event-data() -> ("CtlRef"=w536:refnum<vi>)  [unwired: 1 in, 7 out]
        n167 = call "界面切换.vi"("界面切换队列输入"=w537, "切换界面名称输入"="极限参数界面", "Bool引用句柄"=w536, "状态转移输入"=w538) -> ("布尔"=w534:bool)  [unwired: 7 in]
      }
      event "烧录座设定界面": Mouse Down {
        n168 = event-data() -> ("CtlRef"=w541:refnum<vi>)  [unwired: 1 in, 7 out]
        n169 = call "界面切换.vi"("界面切换队列输入"=w542, "切换界面名称输入"="烧录座设定界面", "Bool引用句柄"=w541, "状态转移输入"=w543) -> ("布尔"=w539:bool)  [unwired: 7 in]
      }
      event Timeout {
        n170 = event-data() -> ()  [unwired: 1 in, 3 out]
      }
      event Panel Close? {
        n171 = event-data() -> ()  [unwired: 1 in, 4 out]
        n172 = Two Button Dialog(message="确定退出程序？" ("消息")) -> (T button?=w547:bool)  [unwired: 2 in]
        n173 = case shown="真" w547 {
          tunnel: [_ TRUE] -> w546
          tunnel: w545 -> [_ w552]
          tunnel: w544 -> [_ w551]
          frame False {
          }
          frame True {
            n174 = call "字符串入队列操作.vi"("字符消息入队列"="退出", "界面切换队列"=w551) -> ()  [unwired: 9 in, 1 out]
            n175 = call "字符串入队列操作.vi"("字符消息入队列"="写退出", "界面切换队列"=w552) -> ()  [unwired: 9 in, 1 out]
          }
        }
        n176 = event-data("Discard?"=TRUE ("放弃？")) -> ()  [unwired: 1 in, 1 out]
      }
    }
  }
  n177 = disable-structure shown="禁用" {
    frame Disabled {
      n178 = call "布尔切换型入队.vi"() -> ()  [unwired: 12 in]
      n179 = call "批量读D+10个+16位.vi"() -> ()  [unwired: 8 in, 4 out]
      n180 = call "批量读D+5个+32位.vi"() -> ()  [unwired: 8 in, 4 out]
      n181 = call "读D16位.vi"() -> ()  [unwired: 8 in, 4 out]
      n182 = call "写D+32位.vi"() -> ()  [unwired: 8 in, 4 out]
      n183 = call "读D32位.vi"() -> ()  [unwired: 9 in, 3 out]
      n184 = call "读触点-8位.vi"() -> ()  [unwired: 8 in, 4 out]
      n185 = call "写触点.vi"() -> ()  [unwired: 9 in, 3 out]
      n186 = call "布尔复位型入队.vi"() -> ()  [unwired: 6 in, 3 out]
      n187 = call "界面切换.vi"() -> ()  [unwired: 11 in, 1 out]
      n188 = call "数值输入窗口.vi"() -> ()  [unwired: 13 in, 3 out]
      n189 = call "数值输入窗口.vi"() -> ()  [unwired: 13 in, 3 out]
      n190 = call "数值输入窗口.vi"() -> ()  [unwired: 13 in, 3 out]
    }
    frame Enabled {
    }
  }
  n191 = disable-structure shown="禁用" {
    frame Disabled {
      n192 = call "读触点-8位.vi"() -> ()  [unwired: 8 in, 4 out]
      n193 = call "写D+32位.vi"() -> ()  [unwired: 8 in, 4 out]
      n194 = call "批量读D+10个+16位.vi"() -> ()  [unwired: 8 in, 4 out]
      n195 = call "写D+16位.vi"() -> ()  [unwired: 7 in, 5 out]
      n196 = call "批量读D+5个+32位.vi"() -> ()  [unwired: 8 in, 4 out]
      n197 = call "字符串入队列操作.vi"() -> ()  [unwired: 11 in, 1 out]
      n198 = call "读D16位.vi"() -> ()  [unwired: 8 in, 4 out]
      n199 = call "读D32位.vi"() -> ()  [unwired: 9 in, 3 out]
      n200 = call "写触点.vi"() -> ()  [unwired: 9 in, 3 out]
      n201 = call "写触点.vi"() -> ()  [unwired: 9 in, 3 out]
    }
    frame Enabled {
    }
  }
  n202 = disable-structure shown="禁用" {
    frame Disabled {
      n203 = for {
        i -> [w557]
        n204 = case shown="9" w557 {
          frame 0, Default {
          }
          frame 1 {
          }
          frame 2 {
          }
          frame 3 {
          }
          frame 4 {
          }
          frame 5 {
          }
          frame 6 {
          }
          frame 7 {
          }
          frame 8 {
          }
          frame 9 {
          }
        }
      }
      n205 = for {
        i -> [w555]
        n206 = case shown="4" w555 {
          frame 0, Default {
          }
          frame 1 {
          }
          frame 2 {
          }
          frame 3 {
          }
          frame 4 {
          }
        }
      }
      n207 = for {
        i -> [w556]
        n208 = case shown="4" w556 {
          frame 0, Default {
          }
          frame 1 {
          }
          frame 2 {
          }
          frame 3 {
          }
          frame 4 {
          }
        }
      }
    }
    frame Enabled {
    }
  }
  n209 = while {
    tunnel: w14 -> [w562]
    tunnel: w13 -> [w561]
    tunnel: w6 -> [w560]
    stop <- TRUE stop-if-true
    n210 = control-ref of="本VI"() -> (w558:refnum<vi>)
    n211 = Release Queue(queue=w560) -> ()  [unwired: 2 in, 3 out]
    n212 = invoke class="VI" method="FP.Close"(reference=w558) -> ()  [unwired: 2 in, 3 out]
    n213 = property on="参数界面" class="Bool"("DisabledEnum"=T3."Enabled" ("禁用")) -> ()  [unwired: 2 in, 2 out]
    "VISA资源名称输出" <- w562
    "错误输出" <- w561
  }
